vi "Z Aux Open Com.vi"(8 "error in (no error)":errorcluster caption="错误输入（无错误）", 10 "phandle":u32, 11 "comid":u32) -> (0 "error out":errorcluster caption="错误输出", 2 "phandle out":u32, 3 "function return":i32)   [LabVIEW 2015, in "zauxdll.lvlib"]
doc: "int32 __stdcall ZAux_OpenCom(uint32 comid, ZMC_HANDLE * phandle);"
uses:
  zauxdll.lvlib
  Radar - 2015 32bit_autoqueue_angle_0319/zauxdll-2014/zauxdll.dll
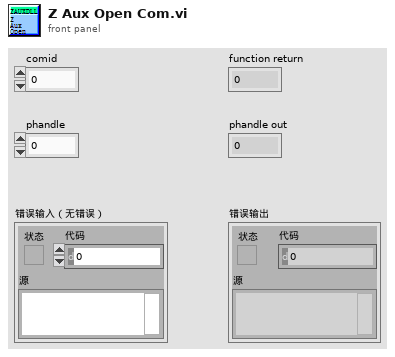
[diagram p1: front panel]
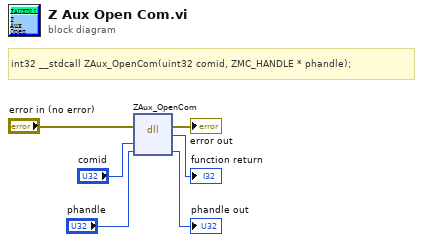
[diagram p0: block diagram]
diagram:
  # "int32 __stdcall ZAux_OpenCom(uint32 comid, ZMC_HANDLE * phandle);"
  n1 = dll-call lib="D:/vicomm case/cub/0717/Radar - 2015 32bit_autoqueue_angle_0319/zauxdll-2014/zauxdll.*" fn="ZAux_OpenCom"(error in="error in (no error)", "comid"="comid", "phandle"="phandle") -> (error out=→"error out":errorcluster, →"function return":i32, "phandle"=→"phandle out":u32)  [unwired: 3 in, 1 out]
